vi "Add State Callback.vi"(7 "Owner":refnum<class>, 8 "error in (no error)":errorcluster, 10 "Callback":refnum<vi>, 11 "Endpoint in":refnum<class "Endpoint.lvclass">) -> (0 "error out":errorcluster, 3 "Endpoint out":refnum<class "Endpoint.lvclass">)   [LabVIEW 2020, in "Stream.lvlib" / "Endpoint.lvclass"]
uses:
  Endpoint.lvclass
  Connection/Connection.lvclass
  State Callback.ctl
  Endpoint.lvclass/Endpoint.ctl
  <vilib>/Utility/error.llb/Error Cluster From Error Code.vi
  <vilib>/ErrorRing/Error Ring.xnode
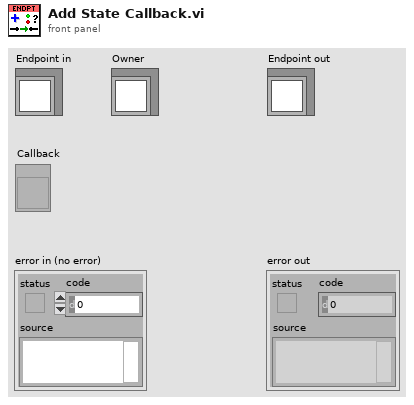
[diagram p1: front panel]
types:
  T1 = typedef "Stream.lvlib/Endpoint.lvclass/State Callback.ctl" = cluster{"Owner":refnum<class>, "VI":refnum<vi>}
  T2 = typedef "Stream.lvlib/Endpoint.lvclass/Ref Data.ctl" = cluster{"URI":refnum<class "URI.lvclass">, "State Callbacks":T1[], "Open":bool, "Mode":T3, "Sniffer Callbacks":T1[]}
  T3 = typedef "Stream.lvlib/Mode.ctl" = enum16{"Raw", "Buffered", "LineTerm"}
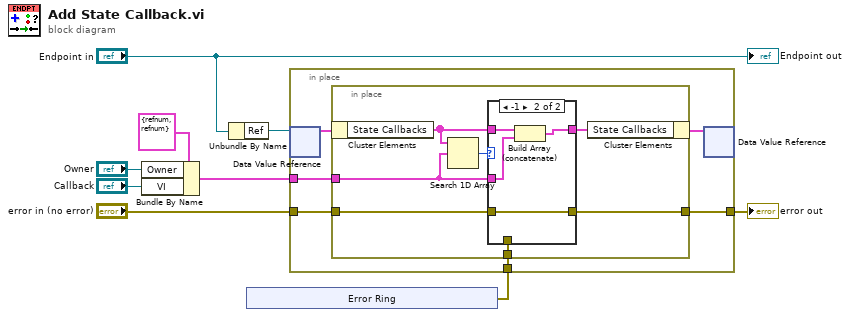
[diagram p0: block diagram]
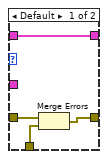
[diagram p2: hidden frame]
diagram:
  n1 = Bundle By Name(cluster=T1 {"Owner"=refnum, "VI"=refnum} ("State Callback"), "Owner"="Owner", "VI"="Callback") -> (w4:T1)
  n2 = Unbundle By Name("Endpoint in") -> ("Ref"=w6:refnum<data-value>)
  n3 = xnode "Error Ring"() -> ("error out"=w2:errorcluster)
  n4 = in-place {
    in-place-border: w4 -> [w13]
    in-place-border: "error in (no error)" -> [w12]
    in-place-border: w2 -> [w11]
    in-place-border: [w10] -> w1
    n5 = in-place-dvr #1(w6) -> (w15:T2)  [unwired: 1 out]
    n6 = in-place {
      in-place-border: w13 -> [w20]
      in-place-border: w12 -> [w18]
      in-place-border: w11 -> [w17]
      in-place-border: [w16] -> w10
      n7 = in-place-cluster #2(w15) -> ("State Callbacks"=w21:T1[])
      n8 = Search 1D Array(1D array=w21, element=w20) -> (index of element=w22:i32)  [unwired: 1 in]
      n9 = case shown="-1" w22 {
        tunnel: w21 -> [w26 w30]
        tunnel: w20 -> [_ w29]
        tunnel: [w26 w28] -> w19
        tunnel: w18 -> [w25 w27]
        tunnel: w17 -> [w24 _]
        tunnel: [w23 w27] -> w16
        frame Default {
          n10 = Merge Errors(w25, w24) -> (w23:errorcluster)
        }
        frame -1 {
          n11 = Build Array (concatenate)(w30, w29) -> (w28:T1[])
        }
      }
      n12 = in-place-cluster #2("State Callbacks"=w19) -> (w14:T2)
    }
    n13 = in-place-dvr #1(w14) -> ()  [unwired: 2 out]
  }
  "error out" <- w1
  "Endpoint out" <- "Endpoint in"
